vi "TCP - Engine.vi"() -> ()   [LabVIEW 2017]
uses:
  SubVIs/Read File.ctl
  Controls/RT- Queue States.ctl
  TCP - Test Settings.ctl
  TCP - Signals.ctl
  TCP - Signal Names.ctl
  Test Execution/Test - Driver control.ctl
  TCP - Driver Control.ctl
  SubVIs/SubVI - Global.vi
panel:
  out "Waveform Chart":u32(graph)
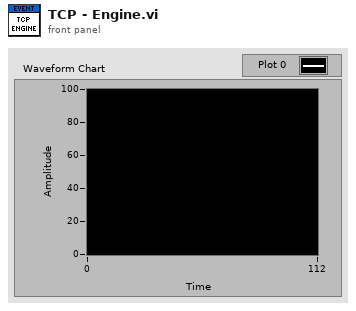
[diagram p1: front panel]
types:
  T1 = typedef "RT- Queue States.ctl" = enum16{"Initialize", "Enqueue", "Enqueue Priority", "Dequeue", "Flush", "Destroy"}
  T2 = typedef "Read File.ctl" = enum16{"Fetch XML", "Open", "Read", "Write", "Close"}
  T3 = typedef "TCP - Test Settings.ctl" = cluster{"Sequence File":string, "Iteration":i32}
  T4 = typedef "TCP - Signals.ctl" = cluster{"Signal":T5, "Value":bool, "Data":variant}
  T5 = typedef "TCP - Signal Names.ctl" = enum16{"Test Running", "Update Sensor Data", "Start Test", "Test Started", "Sequence Complete", "Seuence Aborted", "Abort Test", "Test Settings Updated", "Log Path", "Start Aux Logging", "Stop Aux Logging", "Reset Emergency", "Copy Log File", "Generate Alarm", "Download Files", "Send Test Details"}
  T6 = typedef "Test - Driver control.ctl" = enum16{"Init", "Load Sequence File", "Test Running", "Index Step", "Execute Step", "Send Results", "Sequence Complete", "Sequence Aborted", "Stop Sequence Triggered", "Update Manual Values", "Start Aux Logging", "Stop Aux Logging", "Change Dyno Selection", "Reset Emergency Fault", "Get Dyno Config", "Exit"}
  T7 = cluster{"Test details":cluster{"Furnace":string, "Material":string, "Angle":string, "ID":string, "Flowrate":string, "Test Name":string, "Tested By":string}, "Datalog Duration":dbl}
  T8 = typedef "TCP - Driver Control.ctl" = enum16{"Test Settings", "Boolean Commands", "Test Results", "Send Test Details"}
  T9 = cluster{"Furnace":string, "Material":string, "Angle":string, "ID":string, "Flowrate":string, "Test Name":string, "Tested By":string}
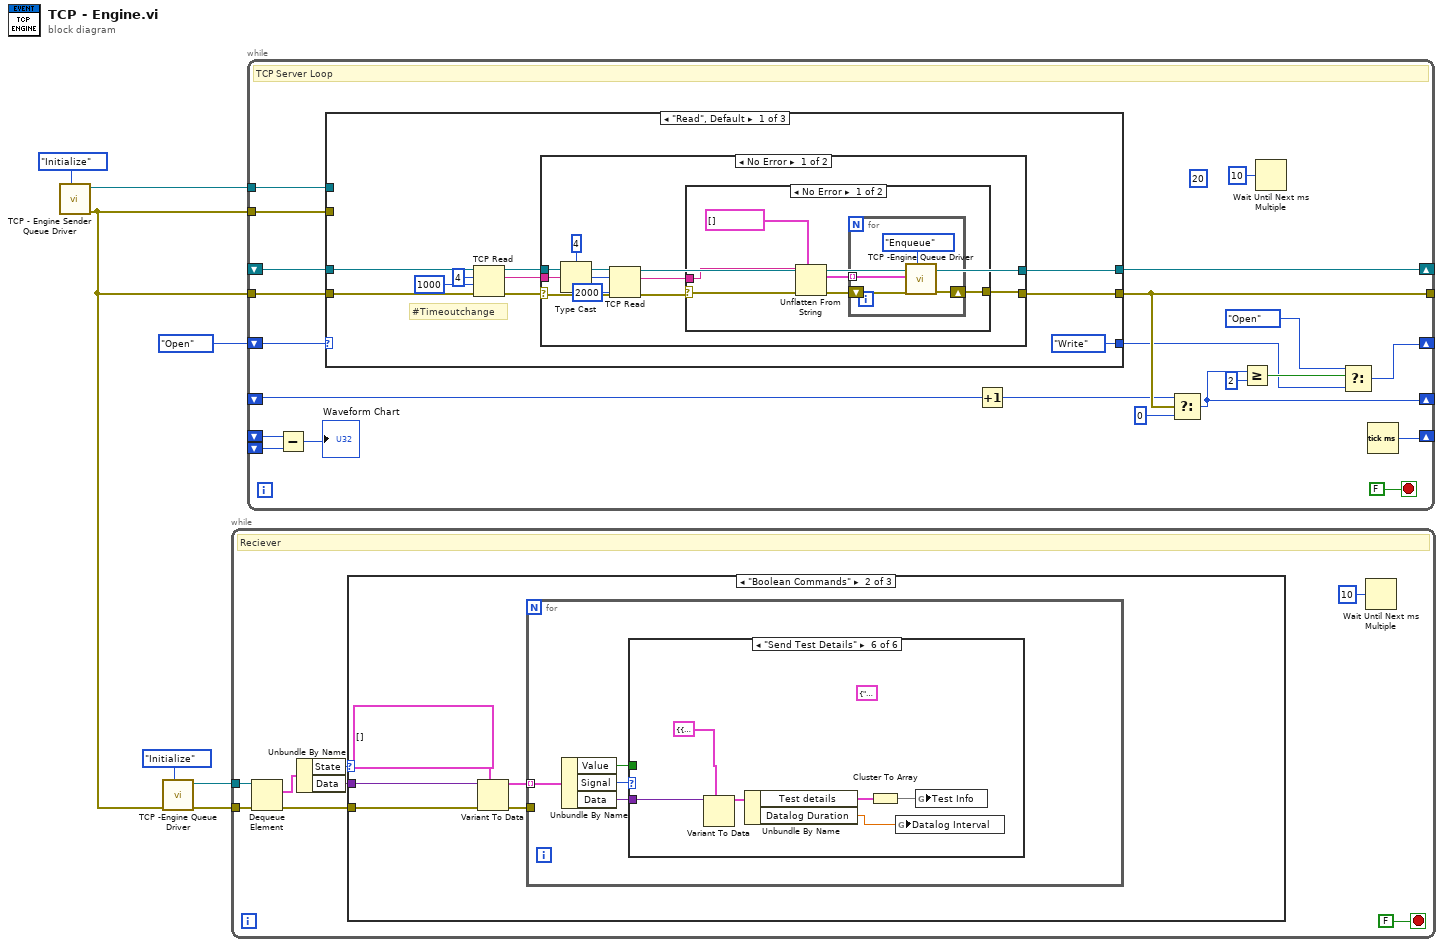
[diagram p0: block diagram]
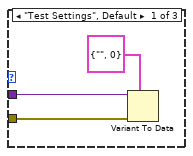
[diagram p2: hidden frame]
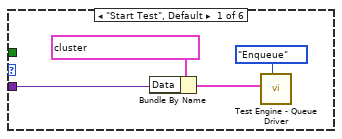
[diagram p3: hidden frame]
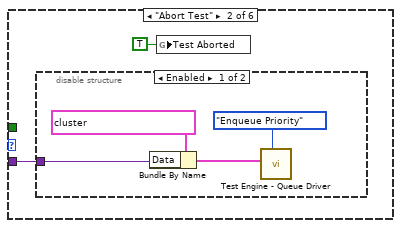
[diagram p4: hidden frame]
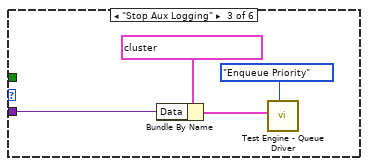
[diagram p6: hidden frame]
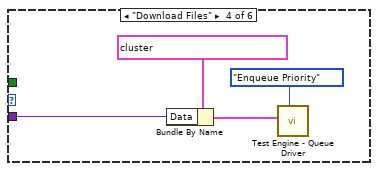
[diagram p7: hidden frame]
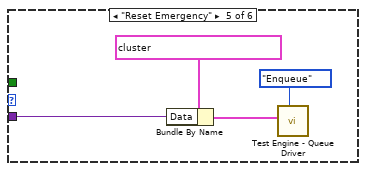
[diagram p8: hidden frame]
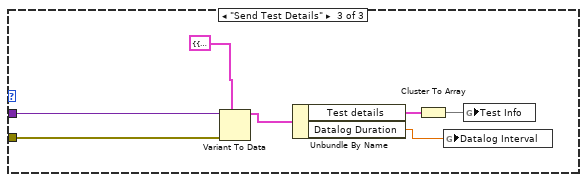
[diagram p9: hidden frame]
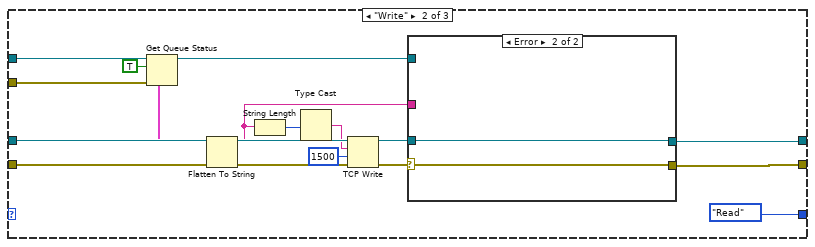
[diagram p12: hidden frame]
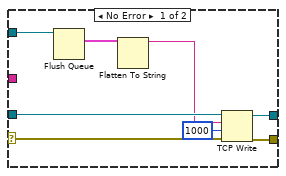
[diagram p13: hidden frame]
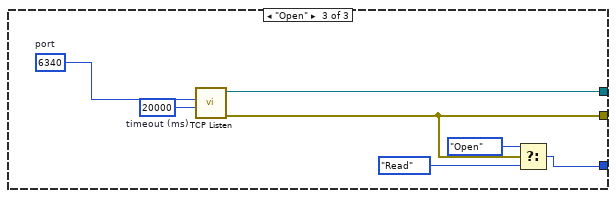
[diagram p14: hidden frame]
diagram:
  n1 = call "TCP - Engine Sender Queue Driver.vi"("Cases"=RT-_Queue_States."Initialize") -> ("error out"=w2:errorcluster, "queue out"=w1:refnum<queue>)  [unwired: 8 in, 1 out]
  n2 = call "TCP -Engine Queue Driver.vi"("Cases"=RT-_Queue_States."Initialize", "error in (no error)"=w2) -> ("error out"=w4:errorcluster, "queue out"=w5:refnum<queue>)  [unwired: 7 in, 1 out]
  n3 = while {
    tunnel: w5 -> [w14]
    tunnel: w4 -> [w15]
    stop <- FALSE stop-if-true
    # "Reciever"
    n4 = Dequeue Element(queue=w14, error in (no error)=w15) -> (element=w12:cluster{"Data":variant, "State":T8}, error out=w13:errorcluster)  [unwired: 1 in, 2 out]
    n5 = Unbundle By Name(w12) -> ("State"=w10:T8, "Data"=w9:variant)
    n6 = case shown="\"Boolean Commands\"" w10 {
      tunnel: w13 -> [w18 w22 w56]
      tunnel: w9 -> [w17 w23 w57]
      frame "Test Settings", Default {
        n7 = Variant To Data(error in=w18, type=T3 {"Sequence File"="", "Iteration"=0}, Variant=w17) -> ()  [unwired: 2 out]
      }
      frame "Boolean Commands" {
        n8 = Variant To Data(error in=w22, type=T4[] [], Variant=w23) -> (data=w20:T4[], error out=w19:errorcluster)
        n9 = for {
          tunnel: w20 -> [w27] mode=indexing
          tunnel: w19 -> [_]
          n10 = Unbundle By Name(w27) -> ("Value"=w25:bool, "Signal"=w26:T5, "Data"=w24:variant)
          n11 = case shown="\"Send Test Details\"" w26 {
            tunnel: w25 -> [_ _ _ _ _ _]
            tunnel: w24 -> [w30 w33 w38 w42 w46 w55]
            frame "Start Test", Default {
              n12 = Bundle By Name(cluster=cluster{"Data":variant, "State":T6} {"Data"=variant, "State"=enum."Load Sequence File"} ("Element In"), "Data"=w30) -> (w28:cluster{"Data":variant, "State":T6})
              n13 = call "Test Engine - Queue Driver.vi"("Cases"=RT-_Queue_States."Enqueue", "Element In"=w28) -> ()  [unwired: 7 in, 3 out]
            }
            frame "Abort Test" {
              n14 = disable-structure shown="Enabled" {
                disable-tunnel: w33 -> [w36 _]
                frame Enabled {
                  n15 = Bundle By Name(cluster=cluster{"Data":variant, "State":T6} {"Data"=variant, "State"=enum."Sequence Aborted"} ("Element In"), "Data"=w36) -> (w34:cluster{"Data":variant, "State":T6})
                  n16 = call "Test Engine - Queue Driver.vi"("Cases"=RT-_Queue_States."Enqueue Priority", "Element In"=w34) -> ()  [unwired: 7 in, 3 out]
                }
                frame Disabled {
                }
              }
              n17 = global write "SubVI - Global.vi" "Test Aborted"(TRUE ("Test Aborted")) -> ()
            }
            frame "Stop Aux Logging" {
              n18 = Bundle By Name(cluster=cluster{"Data":variant, "State":T6} {"Data"=variant, "State"=enum."Stop Aux Logging"} ("Element In"), "Data"=w38) -> (w39:cluster{"Data":variant, "State":T6})
              n19 = call "Test Engine - Queue Driver.vi"("Cases"=RT-_Queue_States."Enqueue Priority", "Element In"=w39) -> ()  [unwired: 7 in, 3 out]
            }
            frame "Download Files" {
              n20 = Bundle By Name(cluster=cluster{"Data":variant, "State":T6} {"Data"=variant, "State"=enum."Change Dyno Selection"} ("Element In"), "Data"=w42) -> (w43:cluster{"Data":variant, "State":T6})
              n21 = call "Test Engine - Queue Driver.vi"("Cases"=RT-_Queue_States."Enqueue Priority", "Element In"=w43) -> ()  [unwired: 7 in, 3 out]
            }
            frame "Reset Emergency" {
              n22 = Bundle By Name(cluster=cluster{"Data":variant, "State":T6} {"Data"=variant, "State"=enum."Reset Emergency Fault"} ("Element In"), "Data"=w46) -> (w47:cluster{"Data":variant, "State":T6})
              n23 = call "Test Engine - Queue Driver.vi"("Cases"=RT-_Queue_States."Enqueue", "Element In"=w47) -> ()  [unwired: 7 in, 3 out]
            }
            frame "Send Test Details" {
              (unwired) T9 {"Furnace"="Furnace A", "Material"="Coke", "Angle"="Multi Angle", "ID"="Trajectory 9", "Flowrate"="Flow", "Test Name"="Coke Burn", "Tested By"="Anirban"} ("Test details")
              n24 = Variant To Data(type=T7 {"Test details"={"Furnace"="Furnace A", "Material"="Aluminium", "Angle"="Multi Angle", "ID"="Trajectory 9", "Flowrate"="Flow", "Test Name"="Coke Burn", "Tested By"="Anirban"}, "Datalog Duration"=0.0}, Variant=w55) -> (data=w52:T7)  [unwired: 1 in, 1 out]
              n25 = Unbundle By Name(w52) -> ("Test details"=w51:T9, "Datalog Duration"=w50:dbl)
              n26 = Cluster To Array(cluster=w51) -> (array=w54:string[])
              n27 = global write "SubVI - Global.vi" "Datalog Interval"(w50) -> ()
              n28 = global write "SubVI - Global.vi" "Test Info"(w54) -> ()
            }
          }
        }
      }
      frame "Send Test Details" {
        n29 = Variant To Data(error in=w56, type=T7 {"Test details"={"Furnace"="Furnace A", "Material"="Aluminium", "Angle"="Multi Angle", "ID"="Trajectory 9", "Flowrate"="Flow", "Test Name"="Coke Burn", "Tested By"="Anirban"}, "Datalog Duration"=0.0}, Variant=w57) -> (data=w60:T7)  [unwired: 1 out]
        n30 = Unbundle By Name(w60) -> ("Test details"=w59:T9, "Datalog Duration"=w58:dbl)
        n31 = Cluster To Array(cluster=w59) -> (array=w62:string[])
        n32 = global write "SubVI - Global.vi" "Datalog Interval"(w58) -> ()
        n33 = global write "SubVI - Global.vi" "Test Info"(w62) -> ()
      }
    }
    n34 = Wait Until Next ms Multiple(millisecond multiple=u32 10) -> ()  [unwired: 1 out]
  }
  n35 = while {
    shift-right: [w83] -> _
    shift-left: _ -> [w82]
    shift-right: [w72] -> _
    shift-left: Read_File."Open" ("R/W") -> [w84]
    shift-right: [w76] -> _
    shift-left: _ -> [w78]
    tunnel: w2 -> [w70]
    tunnel: w1 -> [w69]
    tunnel: w2 -> [w81]
    tunnel: [w80] -> _
    shift-right: [w66] -> _
    shift-left: _ -> [w65]
    shift-left: _ -> [w64]
    stop <- FALSE stop-if-true
    (unwired) u32 20 ("millisecond multiple")
    # "TCP Server Loop"
    n36 = Subtract(x=w65, y=w64) -> (x-y=→"Waveform Chart":u32)
    n37 = case shown="\"Read\", Default" w84 {
      tunnel: [w89 w131 w150] -> w83
      tunnel: [w88 w130 w149] -> w80
      tunnel: w82 -> [w94 w133 _]
      tunnel: w81 -> [w93 w123 _]
      tunnel: [Read_File."Write" ("R/W") Read_File."Read" ("R/W") w146] -> w68
      tunnel: w70 -> [_ w126 _]
      tunnel: w69 -> [_ w127 _]
      frame "Read", Default {
        # "#Timeoutchange"
        n38 = TCP Read(connection ID=w94, bytes to read=4, error in (no error)=w93, 9:1000 ("timeout ms (25000)")) -> (connection ID out=w92:refnum<k5>, data out=w87:string, error out=w85:errorcluster)  [unwired: 1 out]
        n39 = case shown="No Error" w85 {
          selector: w85 -> [w99 w116]
          tunnel: w92 -> [w104 w117]
          tunnel: [w103 w117] -> w89
          tunnel: [w98 w116] -> w88
          tunnel: w87 -> [w101 _]
          frame No Error {
            n40 = Type Cast(type=4 ("bytes to read"), x=w101) -> (*(type *) &x=w100:i32)
            n41 = TCP Read(connection ID=w104, bytes to read=w100, error in (no error)=w99, 9:2000 ("timeout ms (25000)")) -> (connection ID out=w103:refnum<k5>, data out=w97:string, error out=w96:errorcluster)  [unwired: 1 out]
            n42 = case shown="No Error" w96 {
              selector: w96 -> [w107 w115]
              tunnel: w97 -> [w108 _]
              tunnel: [w110 w115] -> w98
              frame No Error {
                n43 = Unflatten From String(type=cluster{"Data":variant, "State":T8}[] [], binary string=w108, error in (no error)=w107) -> (value=w105:cluster{"Data":variant, "State":T8}[], error out=w106:errorcluster)  [unwired: 2 in, 1 out]
                n44 = for {
                  tunnel: w105 -> [w111] mode=indexing
                  shift-right: [w113] -> w110
                  shift-left: w106 -> [w112]
                  n45 = call "TCP -Engine Queue Driver.vi"("Cases"=RT-_Queue_States."Enqueue", "error in (no error)"=w112, "Element In"=w111) -> ("error out"=w113:errorcluster)  [unwired: 6 in, 2 out]
                }
              }
              frame Error {
              }
            }
          }
          frame Error {
          }
        }
      }
      frame "Write" {
        n46 = Get Queue Status(queue=w127, return elements? (F)=TRUE, error in (no error)=w126) -> (queue out=w118:refnum<queue>, elements=w124:cluster{"Data":variant, "State":T8}[])  [unwired: 6 out]
        n47 = Flatten To String(anything=w124, error in (no error)=w123) -> (data string=w119:string, error out=w122:errorcluster)  [unwired: 2 in, 1 out]
        n48 = String Length(string=w119) -> (length=w121:i32)
        n49 = Type Cast(x=w121) -> (*(type *) &x=w120:string)  [unwired: 1 out]
        n50 = TCP Write(connection ID=w133, data in=w120, error in (no error)=w122, 9:1500 ("timeout ms (25000)")) -> (connection ID out=w132:refnum<k5>, error out=w128:errorcluster)  [unwired: 1 out]
        n51 = case shown="Error" w128 {
          selector: w128 -> [w139 w143]
          tunnel: w132 -> [w142 w144]
          tunnel: [w141 w144] -> w131
          tunnel: [w140 w143] -> w130
          tunnel: w119 -> [_ _]
          tunnel: w118 -> [w136 _]
          frame No Error {
            n52 = Flush Queue(queue=w136) -> (remaining elements=w137:cluster{"Data":variant, "State":T8}[])  [unwired: 1 in, 2 out]
            n53 = Flatten To String(anything=w137) -> (data string=w135:string)  [unwired: 3 in, 2 out]
            n54 = TCP Write(connection ID=w142, data in=w135, error in (no error)=w139, 9:1000 ("timeout ms (25000)")) -> (connection ID out=w141:refnum<k5>, error out=w140:errorcluster)  [unwired: 1 out]
          }
          frame Error {
          }
        }
      }
      frame "Open" {
        w145 = u16 6340  # port
        w151 = 20000  # timeout (ms)
        n55 = call <vilib>:"TCP Listen.vi"("timeout ms (wait forever: -1)"=w151, "port"=w145) -> ("error out"=w149:errorcluster, "connection ID"=w150:refnum<k5>)  [unwired: 5 in, 3 out]
        n56 = Select(t=Read_File."Open", s=w149, f=Read_File."Read" ("R/W")) -> (s? t:f=w146:T2)
      }
    }
    n57 = Increment(x=w78) -> (x+1=w77:i32)
    n58 = Select(t=w77, s=w80, f=0) -> (s? t:f=w76:i32)
    n59 = Greater Or Equal?(x=w76, y=2) -> (x >= y?=w73:bool)
    n60 = Wait Until Next ms Multiple(millisecond multiple=u32 10) -> ()  [unwired: 1 out]
    n61 = Select(t=Read_File."Open" ("f"), s=w73, f=w68) -> (s? t:f=w72:T2)
    n62 = Tick Count (ms)() -> (millisecond timer value=w66:u32)
  }
